vi "Gaussian Speed Ramp.vi"(1 "Speed (-1 to 1)":dbl, 2 "lower limit":dbl=0.2 format="%#_13g", 3 "Distance (inches)":dbl, 4 "Current Encoder":dbl, 5 "B Factor":dbl, 6 "Sigma Conversion":dbl=0.3 format="%#_13g") -> (0 "Speed":dbl)   [LabVIEW 2014]
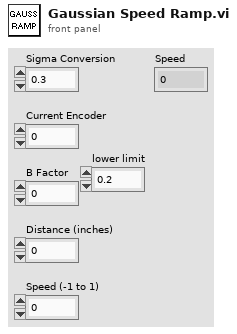
[diagram p1: front panel]
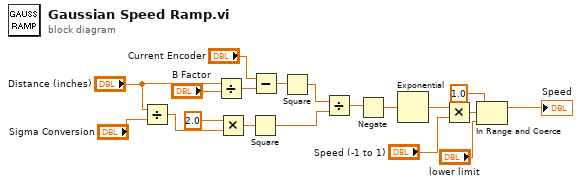
[diagram p0: block diagram]
diagram:
  n1 = Divide(x="Distance (inches)", y="Sigma Conversion") -> (x/y=w11:dbl)
  n2 = Divide(x="Distance (inches)", y="B Factor") -> (x/y=w1:dbl)
  n3 = Multiply(x=2.0 ("y"), y=w11) -> (x*y=w4:dbl)
  n4 = Square(x=w4) -> (x^2=w5:dbl)
  n5 = Subtract(x="Current Encoder", y=w1) -> (x-y=w2:dbl)
  n6 = Square(x=w2) -> (x^2=w6:dbl)
  n7 = Divide(x=w6, y=w5) -> (x/y=w7:dbl)
  n8 = Negate(x=w7) -> (-x=w8:dbl)
  n9 = Exponential(1:w8) -> (0:w9:dbl)
  n10 = Multiply(x=w9, y="Speed (-1 to 1)") -> (x*y=w12:dbl)
  n11 = In Range and Coerce(upper limit=1.0, x=w12, lower limit="lower limit") -> (coerced(x)=→"Speed":dbl)  [unwired: 1 out]
